vi "Load_Diabetes.vi"(8 "error in":errorcluster caption="entrée d'erreur") -> (0 "error out":errorcluster caption="sortie d'erreur", 3 "Tableau":string[][](array[string]))   [LabVIEW 2020]
doc: "Ten baseline variables, age, sex, body mass index, average blood pressure, and six blood serum measurements were obtained for each of n = 442 diabetes patients, as well as the response of interest, a quantitative measure of disease progression one year after baseline.\n\nData Set Characteristics :\n\nNumber of Instances : 442\n\nNumber of Attributes : First 10 columns are numeric predictive values\n\nTarget : Column 11 is a quantitative measure of disease progression one year after baseline\n\nAttribute Information : \n - age in years\n - sex\n - bmi body mass index\n - bp average blood pressure\n - s1 tc, T-Cells (a type of white blood cells)\n - s2 ldl, low-density lipoproteins\n - s3 hdl, high-density lipoproteins\n - s4 tch, thyroid stimulating hormone\n - s5 ltg, lamotrigine\n - s6 glu, blood sugar level\n\nNote : Each of these 10 feature variables have been mean centered and scaled by the standard deviation times n_samples (i.e. the sum of squares of each column totals 1)."
uses:
  Load_Diabetes.lvclass
panel:
  out "Load_Diabetes en sortie":refnum<class "Load_Diabetes.lvclass">
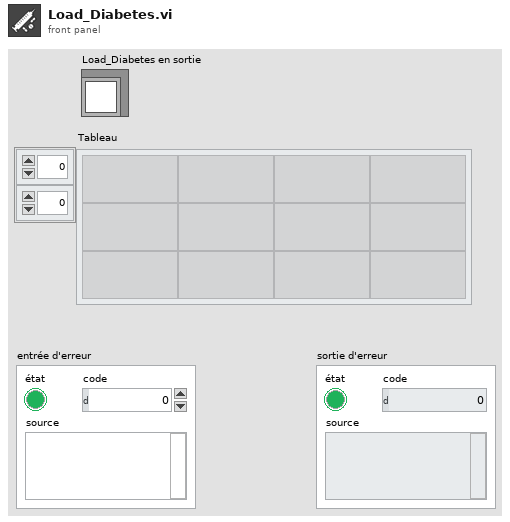
[diagram p1: front panel]
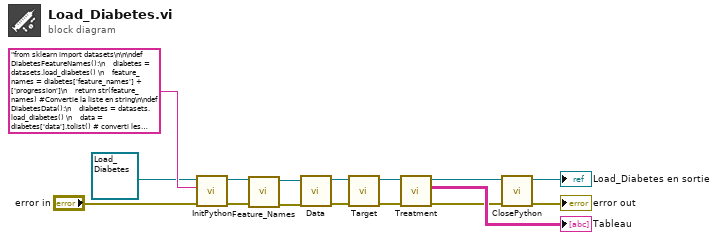
[diagram p0: block diagram]
diagram:
  n1 = call-dynamic "InitPython.vi"("error in (no error)"="error in", "Python Instruction"="from sklearn import datasets\n\n\ndef DiabetesFeatureNames():\n    diabetes = datasets.load_diabetes() \n    feature_names = diabetes['feature_names'] + ['progression']\n    return str(feature_names) #Convertie la liste en string\n\ndef DiabetesData():\n    diabetes = datasets.load_diabetes() \n    data = diabetes['data'].tolist() # converti les datas en une liste\n    return str(data) #Convertie la liste en string\n\ndef DiabetesTarget():\n    diabetes = datasets.load_diabetes() \n    data_target = diabetes['target'].tolist() # converti les datas en une liste\n    return str(data_target) #Convertie la liste en string", "Scikit-learn en entrée"=refnum<class "Load_Diabetes.lvclass"> refnum ("Load_Diabetes.lvclass")) -> ("error out"=w8:errorcluster, "Scikit-learn en sortie"=w9:refnum<class "Load_Diabetes.lvclass">)  [unwired: 7 in]
  n2 = call-dynamic "Feature_Names.vi"("error in (no error)"=w8, "Load_Diabetes en entrée"=w9) -> ("error out"=w6:errorcluster, "Load_Diabetes en sortie"=w7:refnum<class "Load_Diabetes.lvclass">)  [unwired: 8 in]
  n3 = call-dynamic "Data.vi"("error in (no error)"=w6, "Load_Diabetes en entrée"=w7) -> ("error out"=w4:errorcluster, "Load_Diabetes en sortie"=w5:refnum<class "Load_Diabetes.lvclass">)  [unwired: 8 in]
  n4 = call-dynamic "Target.vi"("error in (no error)"=w4, "Load_Diabetes en entrée"=w5) -> ("error out"=w2:errorcluster, "Load_Diabetes en sortie"=w3:refnum<class "Load_Diabetes.lvclass">)  [unwired: 8 in]
  n5 = call-dynamic "Treatment.vi"("error in (no error)"=w2, "Load_Diabetes en entrée"=w3) -> ("error out"=w10:errorcluster, "Tableau"=→"Tableau":string[][], "Load_Diabetes en sortie"=w11:refnum<class "Load_Diabetes.lvclass">)  [unwired: 7 in]
  n6 = call-dynamic "ClosePython.vi"("error in (no error)"=w10, "Scikit-learn en entrée"=w11) -> ("error out"=→"error out":errorcluster, "Scikit-learn en sortie"=→"Load_Diabetes en sortie":refnum<class "Load_Diabetes.lvclass">)  [unwired: 8 in]
